vi "语句解析测试.vi"() -> ()   [LabVIEW 2019, in "test.lvlib"]
uses:
  test.lvlib
  lib/QDInstrument.dll
  SubVI.lvlib
panel:
  out "数字 8":dbl
  out "数字 7":dbl
  out "数字 6":dbl
  out "数字 5":dbl
  out "数字 4":dbl
  out "数字 3":dbl
  out "数字 2":dbl
  out "数字":dbl
  out "Instrument Ref":refnum<k24>
  out "项名":string[](array[string])
  in  "列表框":i32(listbox)
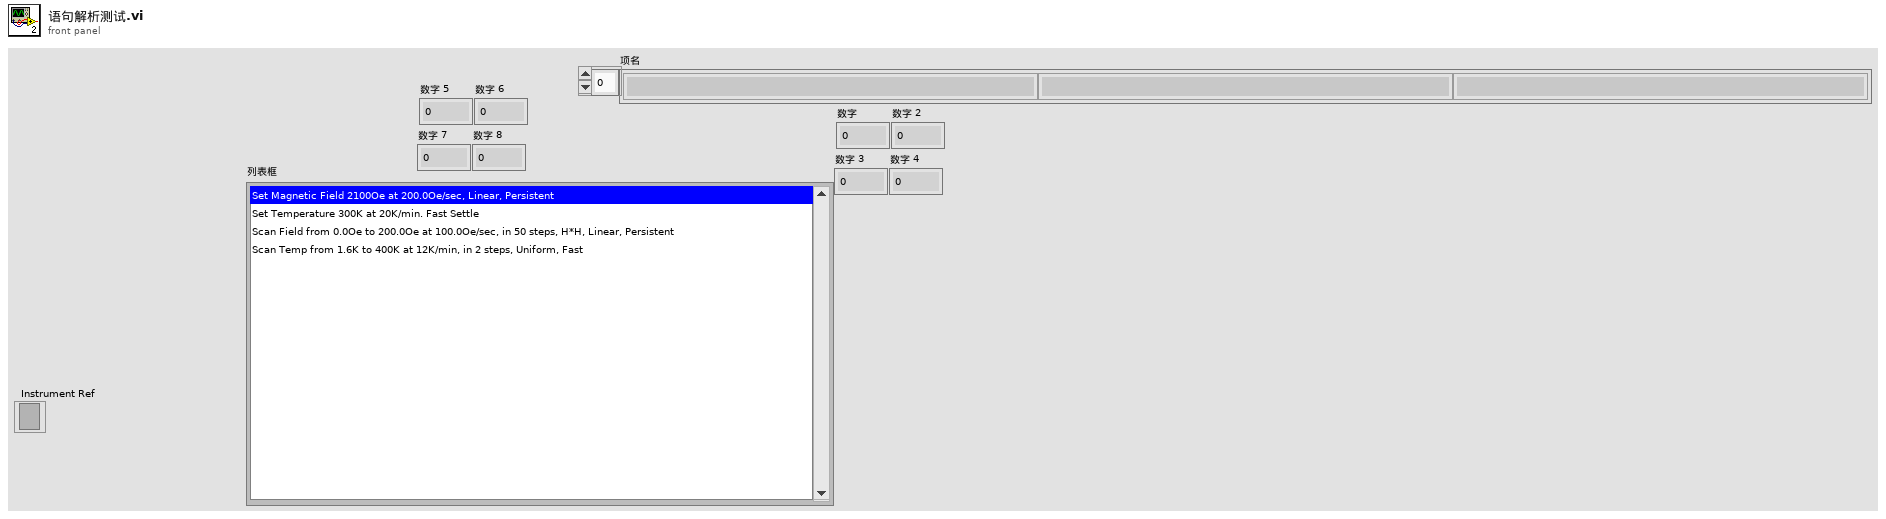
[diagram p1: front panel]
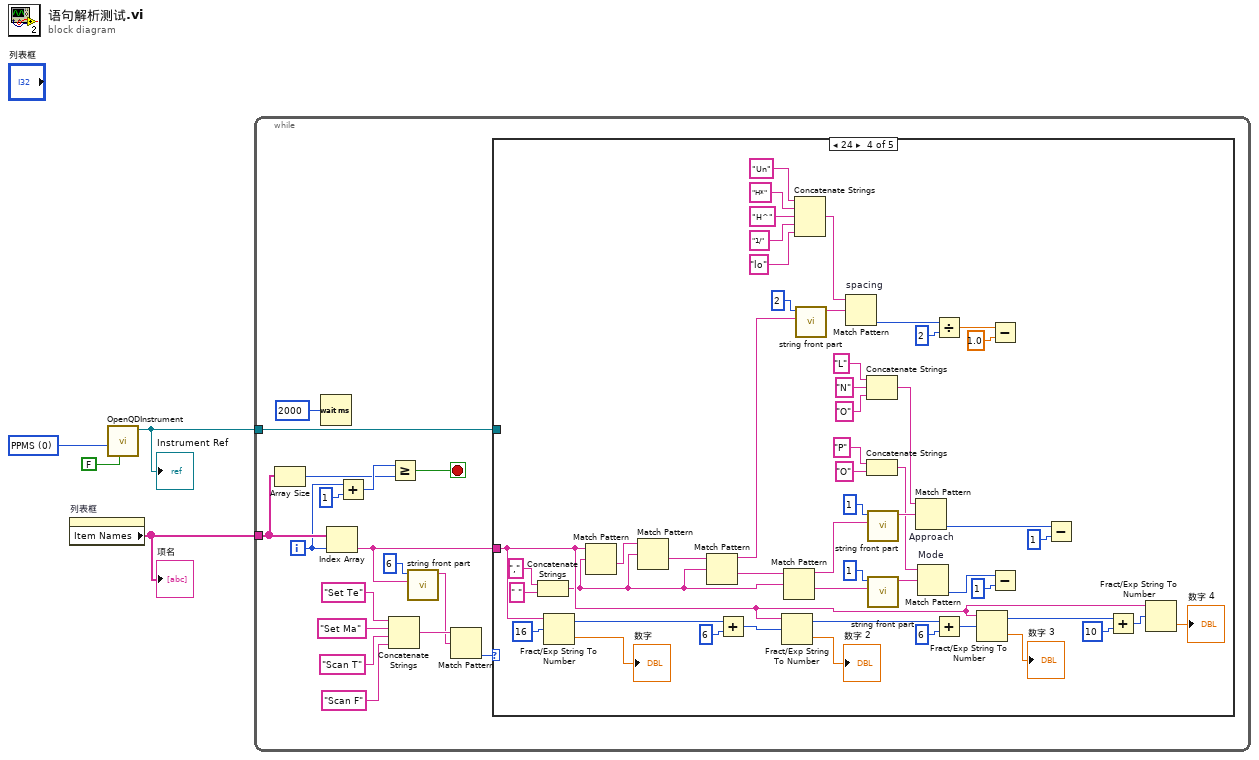
[diagram p0: block diagram]
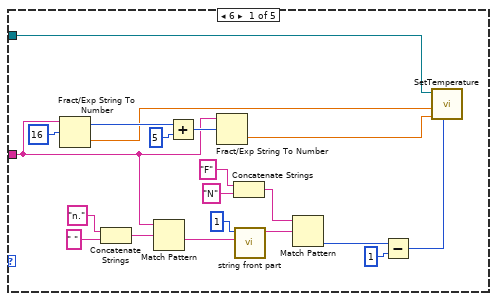
[diagram p2: hidden frame]
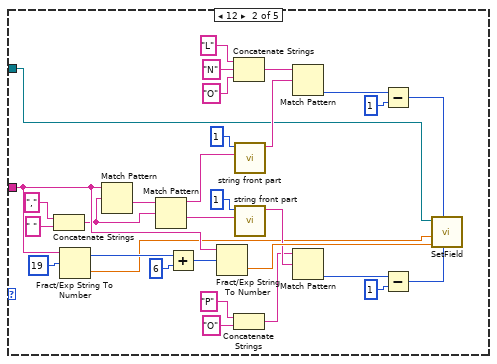
[diagram p3: hidden frame]
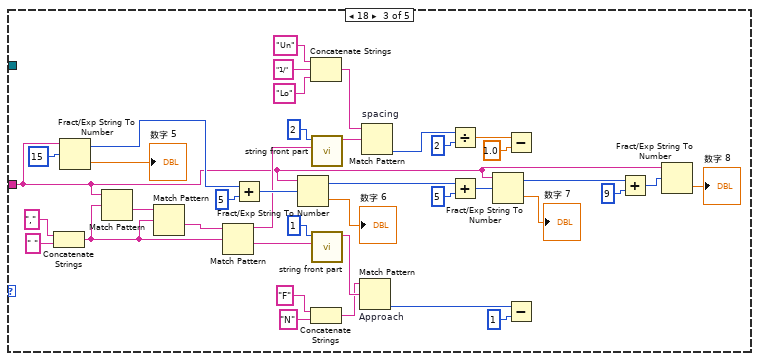
[diagram p4: hidden frame]
diagram:
  w3 = 0 items=["PPMS", "VersaLab", "DynaCool", "SVSM"] ("Instrument Type")
  n1 = property on="列表框" class="LstBox (严格)"() -> ("Item Names"=w4:string[])  [unwired: 2 in, 2 out]
  "项名" <- w4
  n2 = call "OpenQDInstrument.vi"("Remote"=FALSE, "Instrument Type"=w3) -> ("Instrument Ref"=w1:refnum<k24>)  [unwired: 6 in, 1 out]
  "Instrument Ref" <- w1
  n3 = while {
    tunnel: w4 -> [w21]
    tunnel: w1 -> [w5]
    i -> [w20]
    stop <- w16 stop-if-true
    n4 = Array Size(array=w21) -> (size(s)=w17:i32)
    n5 = Wait (ms)(milliseconds to wait=u32 2000 ("等待时间（毫秒）")) -> ()  [unwired: 1 out]
    n6 = Index Array(array=w21, index=w20) -> (element=w6:string)
    n7 = Add(x=w20, y=1) -> (x+y=w18:i32)
    n8 = Concatenate Strings("Set Te" ("字符串"), "Set Ma" ("字符串"), "Scan T" ("字符串"), "Scan F" ("字符串")) -> (w13:string)
    n9 = Greater Or Equal?(x=w18, y=w17) -> (x >= y?=w16:bool)
    n10 = call "string front part.vi"("字符串"=w6, "偏移量(0)"=6) -> ("result string"=w8:string)  [unwired: 9 in]
    n11 = Match Pattern(string=w13, regular expression=w8) -> (offset past match=w7:i32)  [unwired: 1 in, 3 out]
    n12 = case shown="24" w7 {
      tunnel: w6 -> [w30 w68 w74 w135 _]
      tunnel: w5 -> [w25 w45 _ _ _]
      frame 6 {
        n13 = Fract/Exp String To Number(string=w30, offset=16 ("偏移量")) -> (offset past number=w40:i32, number=w28:dbl)  [unwired: 2 in]
        n14 = Concatenate Strings("n." ("正则表达式"), " " ("字符串")) -> (w22:string)
        n15 = Match Pattern(string=w30, regular expression=w22) -> (after substring=w29:string)  [unwired: 1 in, 3 out]
        n16 = Add(x=w40, y=5) -> (x+y=w39:i32)
        n17 = Fract/Exp String To Number(string=w30, offset=w39) -> (number=w27:dbl)  [unwired: 2 in, 1 out]
        n18 = Concatenate Strings("F" ("字符串"), "N" ("字符串")) -> (w33:string)
        n19 = call "string front part.vi"("字符串"=w29, "偏移量(0)"=1) -> ("result string"=w36:string)  [unwired: 9 in]
        n20 = Match Pattern(string=w33, regular expression=w36) -> (offset past match=w32:i32)  [unwired: 1 in, 3 out]
        n21 = Subtract(x=w32, y=1) -> (x-y=w26:i32)
        n22 = call "SetTemperature.vi"("Approach"=w26, "Rate"=w27, "Temperature"=w28, "Instrument Ref In"=w25) -> ()  [unwired: 3 in, 3 out]
      }
      frame 12 {
        n23 = Concatenate Strings("," ("字符串"), " " ("字符串")) -> (w42:string)
        n24 = Fract/Exp String To Number(string=w68, offset=19 ("偏移量")) -> (offset past number=w70:i32, number=w46:dbl)  [unwired: 2 in]
        n25 = Match Pattern(string=w68, regular expression=w42) -> (after substring=w72:string)  [unwired: 1 in, 3 out]
        n26 = Match Pattern(string=w72, regular expression=w42) -> (before substring=w51:string, after substring=w50:string)  [unwired: 1 in, 2 out]
        n27 = Add(x=w70, y=6) -> (x+y=w69:i32)
        n28 = Fract/Exp String To Number(string=w68, offset=w69) -> (number=w67:dbl)  [unwired: 2 in, 1 out]
        n29 = Concatenate Strings("L" ("字符串"), "N" ("字符串"), "O" ("字符串")) -> (w60:string)
        n30 = Concatenate Strings("P" ("字符串"), "O" ("字符串")) -> (w53:string)
        n31 = call "string front part.vi"("字符串"=w51, "偏移量(0)"=1) -> ("result string"=w64:string)  [unwired: 9 in]
        n32 = call "string front part.vi"("字符串"=w50, "偏移量(0)"=1) -> ("result string"=w56:string)  [unwired: 9 in]
        n33 = Match Pattern(string=w60, regular expression=w64) -> (offset past match=w59:i32)  [unwired: 1 in, 3 out]
        n34 = Match Pattern(string=w53, regular expression=w56) -> (offset past match=w52:i32)  [unwired: 1 in, 3 out]
        n35 = Subtract(x=w59, y=1) -> (x-y=w47:i32)
        n36 = Subtract(x=w52, y=1) -> (x-y=w48:i32)
        n37 = call "SetField.vi"("Mode"=w48, "Approach"=w47, "Rate"=w67, "Field"=w46, "Instrument Ref In"=w45) -> ()  [unwired: 2 in, 3 out]
      }
      frame 18 {
        n38 = Concatenate Strings("," ("字符串"), " " ("字符串")) -> (w91:string)
        n39 = Fract/Exp String To Number(string=w74, offset=15 ("偏移量")) -> (offset past number=w109:i32, number=→"数字 5":dbl)  [unwired: 2 in]
        n40 = Match Pattern(string=w74, regular expression=w91) -> (after substring=w111:string)  [unwired: 1 in, 3 out]
        n41 = Match Pattern(string=w111, regular expression=w91) -> (after substring=w92:string)  [unwired: 1 in, 3 out]
        n42 = Match Pattern(string=w92, regular expression=w91) -> (before substring=w90:string, after substring=w73:string)  [unwired: 1 in, 2 out]
        n43 = Add(x=w109, y=5) -> (x+y=w108:i32)
        n44 = Fract/Exp String To Number(string=w74, offset=w108) -> (offset past number=w97:i32, number=→"数字 6":dbl)  [unwired: 2 in]
        n45 = Concatenate Strings("Un" ("字符串"), "1/" ("字符串"), "Lo" ("字符串")) -> (w84:string)
        n46 = Concatenate Strings("F" ("字符串"), "N" ("字符串")) -> (w102:string)
        n47 = call "string front part.vi"("字符串"=w90, "偏移量(0)"=2) -> ("result string"=w88:string)  [unwired: 9 in]
        n48 = call "string front part.vi"("字符串"=w73, "偏移量(0)"=1) -> ("result string"=w105:string)  [unwired: 9 in]
        n49 = Match Pattern "Approach"(string=w102, regular expression=w105) -> (offset past match=w101:i32)  [unwired: 1 in, 3 out]
        n50 = Match Pattern "spacing"(string=w84, regular expression=w88) -> (offset past match=w83:i32)  [unwired: 1 in, 3 out]
        n51 = Divide(x=w83, y=2) -> (x/y=w81:dbl)
        n52 = Add(x=w97, y=5) -> (x+y=w95:i32)
        n53 = Fract/Exp String To Number(string=w74, offset=w95) -> (offset past number=w75:i32, number=→"数字 7":dbl)  [unwired: 2 in]
        n54 = Subtract(x=w81, y=1.0) -> ()  [unwired: 1 out]
        n55 = Subtract(x=w101, y=1) -> ()  [unwired: 1 out]
        n56 = Add(x=w75, y=9) -> (x+y=w93:i32)
        n57 = Fract/Exp String To Number(string=w74, offset=w93) -> (number=→"数字 8":dbl)  [unwired: 2 in, 1 out]
      }
      frame 24 {
        n58 = Concatenate Strings("," ("字符串"), " " ("字符串")) -> (w114:string)
        n59 = Fract/Exp String To Number(string=w135, offset=16 ("偏移量")) -> (offset past number=w160:i32, number=→"数字":dbl)  [unwired: 2 in]
        n60 = Match Pattern(string=w135, regular expression=w114) -> (after substring=w162:string)  [unwired: 1 in, 3 out]
        n61 = Match Pattern(string=w162, regular expression=w114) -> (after substring=w134:string)  [unwired: 1 in, 3 out]
        n62 = Match Pattern(string=w134, regular expression=w114) -> (before substring=w133:string, after substring=w115:string)  [unwired: 1 in, 2 out]
        n63 = Add(x=w160, y=6) -> (x+y=w159:i32)
        n64 = Fract/Exp String To Number(string=w135, offset=w159) -> (offset past number=w140:i32, number=→"数字 2":dbl)  [unwired: 2 in]
        n65 = Match Pattern(string=w115, regular expression=w114) -> (before substring=w113:string, after substring=w112:string)  [unwired: 1 in, 2 out]
        n66 = Concatenate Strings("Un" ("字符串"), "H*" ("字符串"), "H^" ("字符串"), "1/" ("字符串"), "lo" ("字符串")) -> (w125:string)
        n67 = call "string front part.vi"("字符串"=w133, "偏移量(0)"=2) -> ("result string"=w131:string)  [unwired: 9 in]
        n68 = Match Pattern "spacing"(string=w125, regular expression=w131) -> (offset past match=w124:i32)  [unwired: 1 in, 3 out]
        n69 = Concatenate Strings("L" ("字符串"), "N" ("字符串"), "O" ("字符串")) -> (w152:string)
        n70 = Concatenate Strings("P" ("字符串"), "O" ("字符串")) -> (w145:string)
        n71 = call "string front part.vi"("字符串"=w113, "偏移量(0)"=1) -> ("result string"=w156:string)  [unwired: 9 in]
        n72 = call "string front part.vi"("字符串"=w112, "偏移量(0)"=1) -> ("result string"=w148:string)  [unwired: 9 in]
        n73 = Match Pattern "Approach"(string=w152, regular expression=w156) -> (offset past match=w151:i32)  [unwired: 1 in, 3 out]
        n74 = Match Pattern "Mode"(string=w145, regular expression=w148) -> (offset past match=w144:i32)  [unwired: 1 in, 3 out]
        n75 = Divide(x=w124, y=2) -> (x/y=w122:dbl)
        n76 = Add(x=w140, y=6) -> (x+y=w138:i32)
        n77 = Fract/Exp String To Number(string=w135, offset=w138) -> (offset past number=w116:i32, number=→"数字 3":dbl)  [unwired: 2 in]
        n78 = Subtract(x=w122, y=1.0) -> ()  [unwired: 1 out]
        n79 = Subtract(x=w144, y=1) -> ()  [unwired: 1 out]
        n80 = Subtract(x=w151, y=1) -> ()  [unwired: 1 out]
        n81 = Add(x=w116, y=10) -> (x+y=w136:i32)
        n82 = Fract/Exp String To Number(string=w135, offset=w136) -> (number=→"数字 4":dbl)  [unwired: 2 in, 1 out]
      }
      frame -1, Default {
      }
    }
  }
